vi "Distance To Steps.vi"(1 "Desired Distance (mm)":dbl) -> (0 "Number of Steps":string)   [LabVIEW 2020]
doc: "Converts the input of millimetres into number of steps for the stepper motors. \nConversion factor of 5000 Steps --> 1mm\n\nArgs:\n\nDesired Distance (mm): Any dimension (e.g. width of the tank) set by the user in form of an integer.\n\nReturns:\n\nNumber of Steps: Form of a string as string concatuation needs to occur for the ASCII command that will be sent to the scanning rig controller"
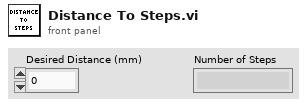
[diagram p1: front panel]
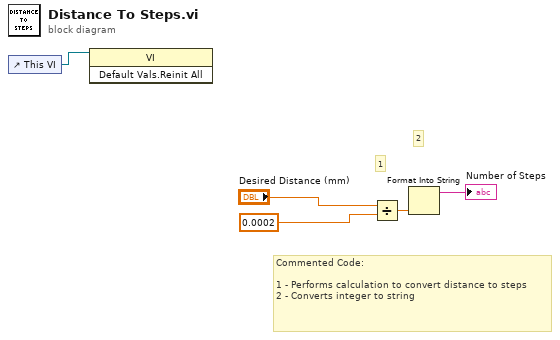
[diagram p0: block diagram]
diagram:
  # "2"
  # "1"
  # "Commented Code:\n\n1 - Performs calculation to convert distance to steps\n2 - Converts integer to string"
  n1 = control-ref of="This VI"() -> (w1:refnum<vi>)
  n2 = invoke class="VI" method="Default Vals.Reinit All"(reference=w1) -> ()  [unwired: 2 in, 3 out]
  n3 = Divide(x="Desired Distance (mm)", y=0.0002) -> (x/y=w3:dbl)
  n4 = Format Into String(w3) -> (resulting string=→"Number of Steps":string)  [unwired: 3 in, 1 out]
